vi "Periodic Tasks.vi"(8 "error in":errorcluster) -> ()   [LabVIEW 2020]
doc: "This VI runs in parallel to other tasks. It can contain as many user-defined periodic loops as you need. These can carry out PID or other sorts of timed response."
uses:
  <vilib>/Rock Robotics/WPI/ThirdParty/Phoenix-LabVIEW/Motor Controller/Controls/CTRE_Phoenix_MotorControl_ControlMode.ctl
  <vilib>/Rock Robotics/WPI/DriverStation/WPI_DriverStationRobotMode2.ctl
  <vilib>/Rock Robotics/WPI/Utilities/WPI_GetSetVariantRefNum.vi
  <vilib>/Rock Robotics/Network Tables/NT Write Numeric Array.vi
  Robot Global Data.vi
  <vilib>/Rock Robotics/Network Tables/NT Write Boolean Array.vi
  <vilib>/Rock Robotics/Network Tables/NT Write Number.vi
  <vilib>/Rock Robotics/Network Tables/NT Write Boolean.vi
  <vilib>/Rock Robotics/WPI/RobotDrive/WPI_RobotDriveMecanumDrive_Cartesian.vi
panel:
  out "Slow Speed ON":bool
  out "Backwards ON":bool
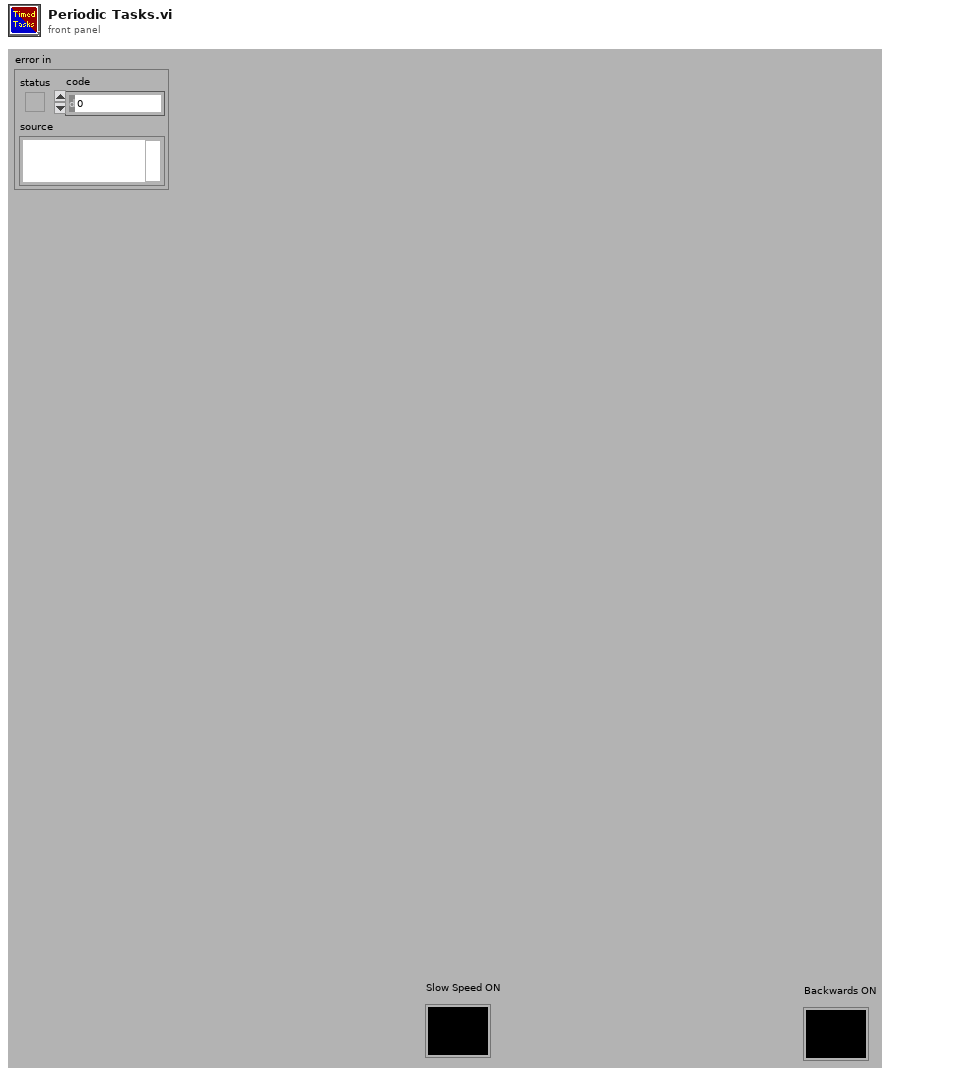
[diagram p1: front panel]
types:
  T1 = typedef "WPI_MotorControlDeviceRef.ctl" = cluster{"DeviceStatus":errorcluster, "Type":T2, "PWM":cluster{"PWM Channel":T3, "DeadBand":T4}, "CAN":cluster{"Device Number":u8, "SetOutput VI Ref":variant, "GetOutput VI Ref":variant, "Enable VI Ref":variant, "Disable VI Ref":variant, "Data":variant}, "Invert":bool, "DIO PWM":cluster{"PWM \"Enable\" Channel":T3, "DIOChannel":T5, "PWM Rate":dbl}}
  T2 = typedef "WPI_MotorControlType.ctl" = enum16{"PWM", "CAN", "DIO PWM"}
  T3 = typedef "FPGA_DIOPWMChannel.ctl" = enum8{"PWM 0", "PWM 1", "PWM 2", "PWM 3", "PWM 4", "PWM 5", "PWM 6", "PWM 7", "PWM 8", "PWM 9", "PWM MXP 0", "PWM MXP 1", "PWM MXP 2", "PWM MXP 3", "PWM MXP 4", "PWM MXP 5", "PWM MXP 6", "PWM MXP 7", "PWM MXP 8", "PWM MXP 9", "Invalid"}
  T4 = typedef "WPI_PWMDeadband.ctl" = cluster{"Name":string, "maxPositivePwm":i32, "minPositivePwm":i32, "centerPwm":i32, "maxNegativePwm":i32, "minNegativePwm":i32, "angularRange":u16}
  T5 = typedef "FPGA_DIOChannel.ctl" = enum8{"DIO 0", "DIO 1", "DIO 2", "DIO 3", "DIO 4", "DIO 5", "DIO 6", "DIO 7", "DIO 8", "DIO 9", "DIO MXP 0", "DIO MXP 1", "DIO MXP 2", "DIO MXP 3", "DIO MXP 4", "DIO MXP 5", "DIO MXP 6", "DIO MXP 7", "DIO MXP 8", "DIO MXP 9", "DIO MXP 10", "DIO MXP 11", "DIO MXP 12", "DIO MXP 13", "DIO MXP 14", "DIO MXP 15", "SPI Port CS1", "SPI Port CS2", "SPI Port CS3", "SPI Port MISO", "SPI Port MOSI", "Invalid"}
  T6 = typedef "WPI_JoystickDevRef.ctl" = cluster{"Device":T7}
  T7 = typedef "WPI_JoystickDeviceEnum.ctl" = enum16{"USB 0", "USB 1", "USB 2", "USB 3", "USB 4", "USB 5"}
  T8 = typedef "WPI_RobotDriveDevRef.ctl" = cluster{"DevStatus":errorcluster, "Motors[]":T1[], "Square Inputs":bool, "Max Output":dbl}
  T9 = typedef "WPI_ServoDeviceRef.ctl" = cluster{"DeviceStatus":errorcluster, "PWM Channel":T3, "DeadBand":T4}
  T10 = typedef "WPI_DriverStationRobotMode2.ctl" = enum16{"Autonomous Disabled", "Autonomous Enabled", "Teleop Disabled", "Teleop Enabled", "Disconnected", "Finish", "Test Disabled", "Test Enabled", "Emergency Stopped"}
  T11 = typedef "CTRE_Phoenix_MotorControl_ControlMode.ctl" = u16
  T12 = typedef "WPI_GyroDevRef.ctl" = cluster{"DevStatus":errorcluster, "Analog Channel":T13, "Gain (VoltsPerDegree/Second)":dbl, "Gyro Type":enum16{"Analog", "XRS450"}, "Handle":i32, "SPI Bus":T14, "Device Found":bool, "Sample Rate":dbl, "Calibrate On Open":bool, "Offset":dbl}
  T13 = typedef "FPGA_AIChannel.ctl" = enum8{"AI 0", "AI 1", "AI 2", "AI 3", "AI MXP 0", "AI MXP 1", "AI MXP 2", "AI MXP 3", "Invalid"}
  T14 = typedef "spi_bus.ctl" = enum16{"SPI On-Board, CS0", "SPI On-Board, CS1", "SPI On-Board, CS2", "SPI On-Board, CS3", "SPI MXP", "Invalid"}
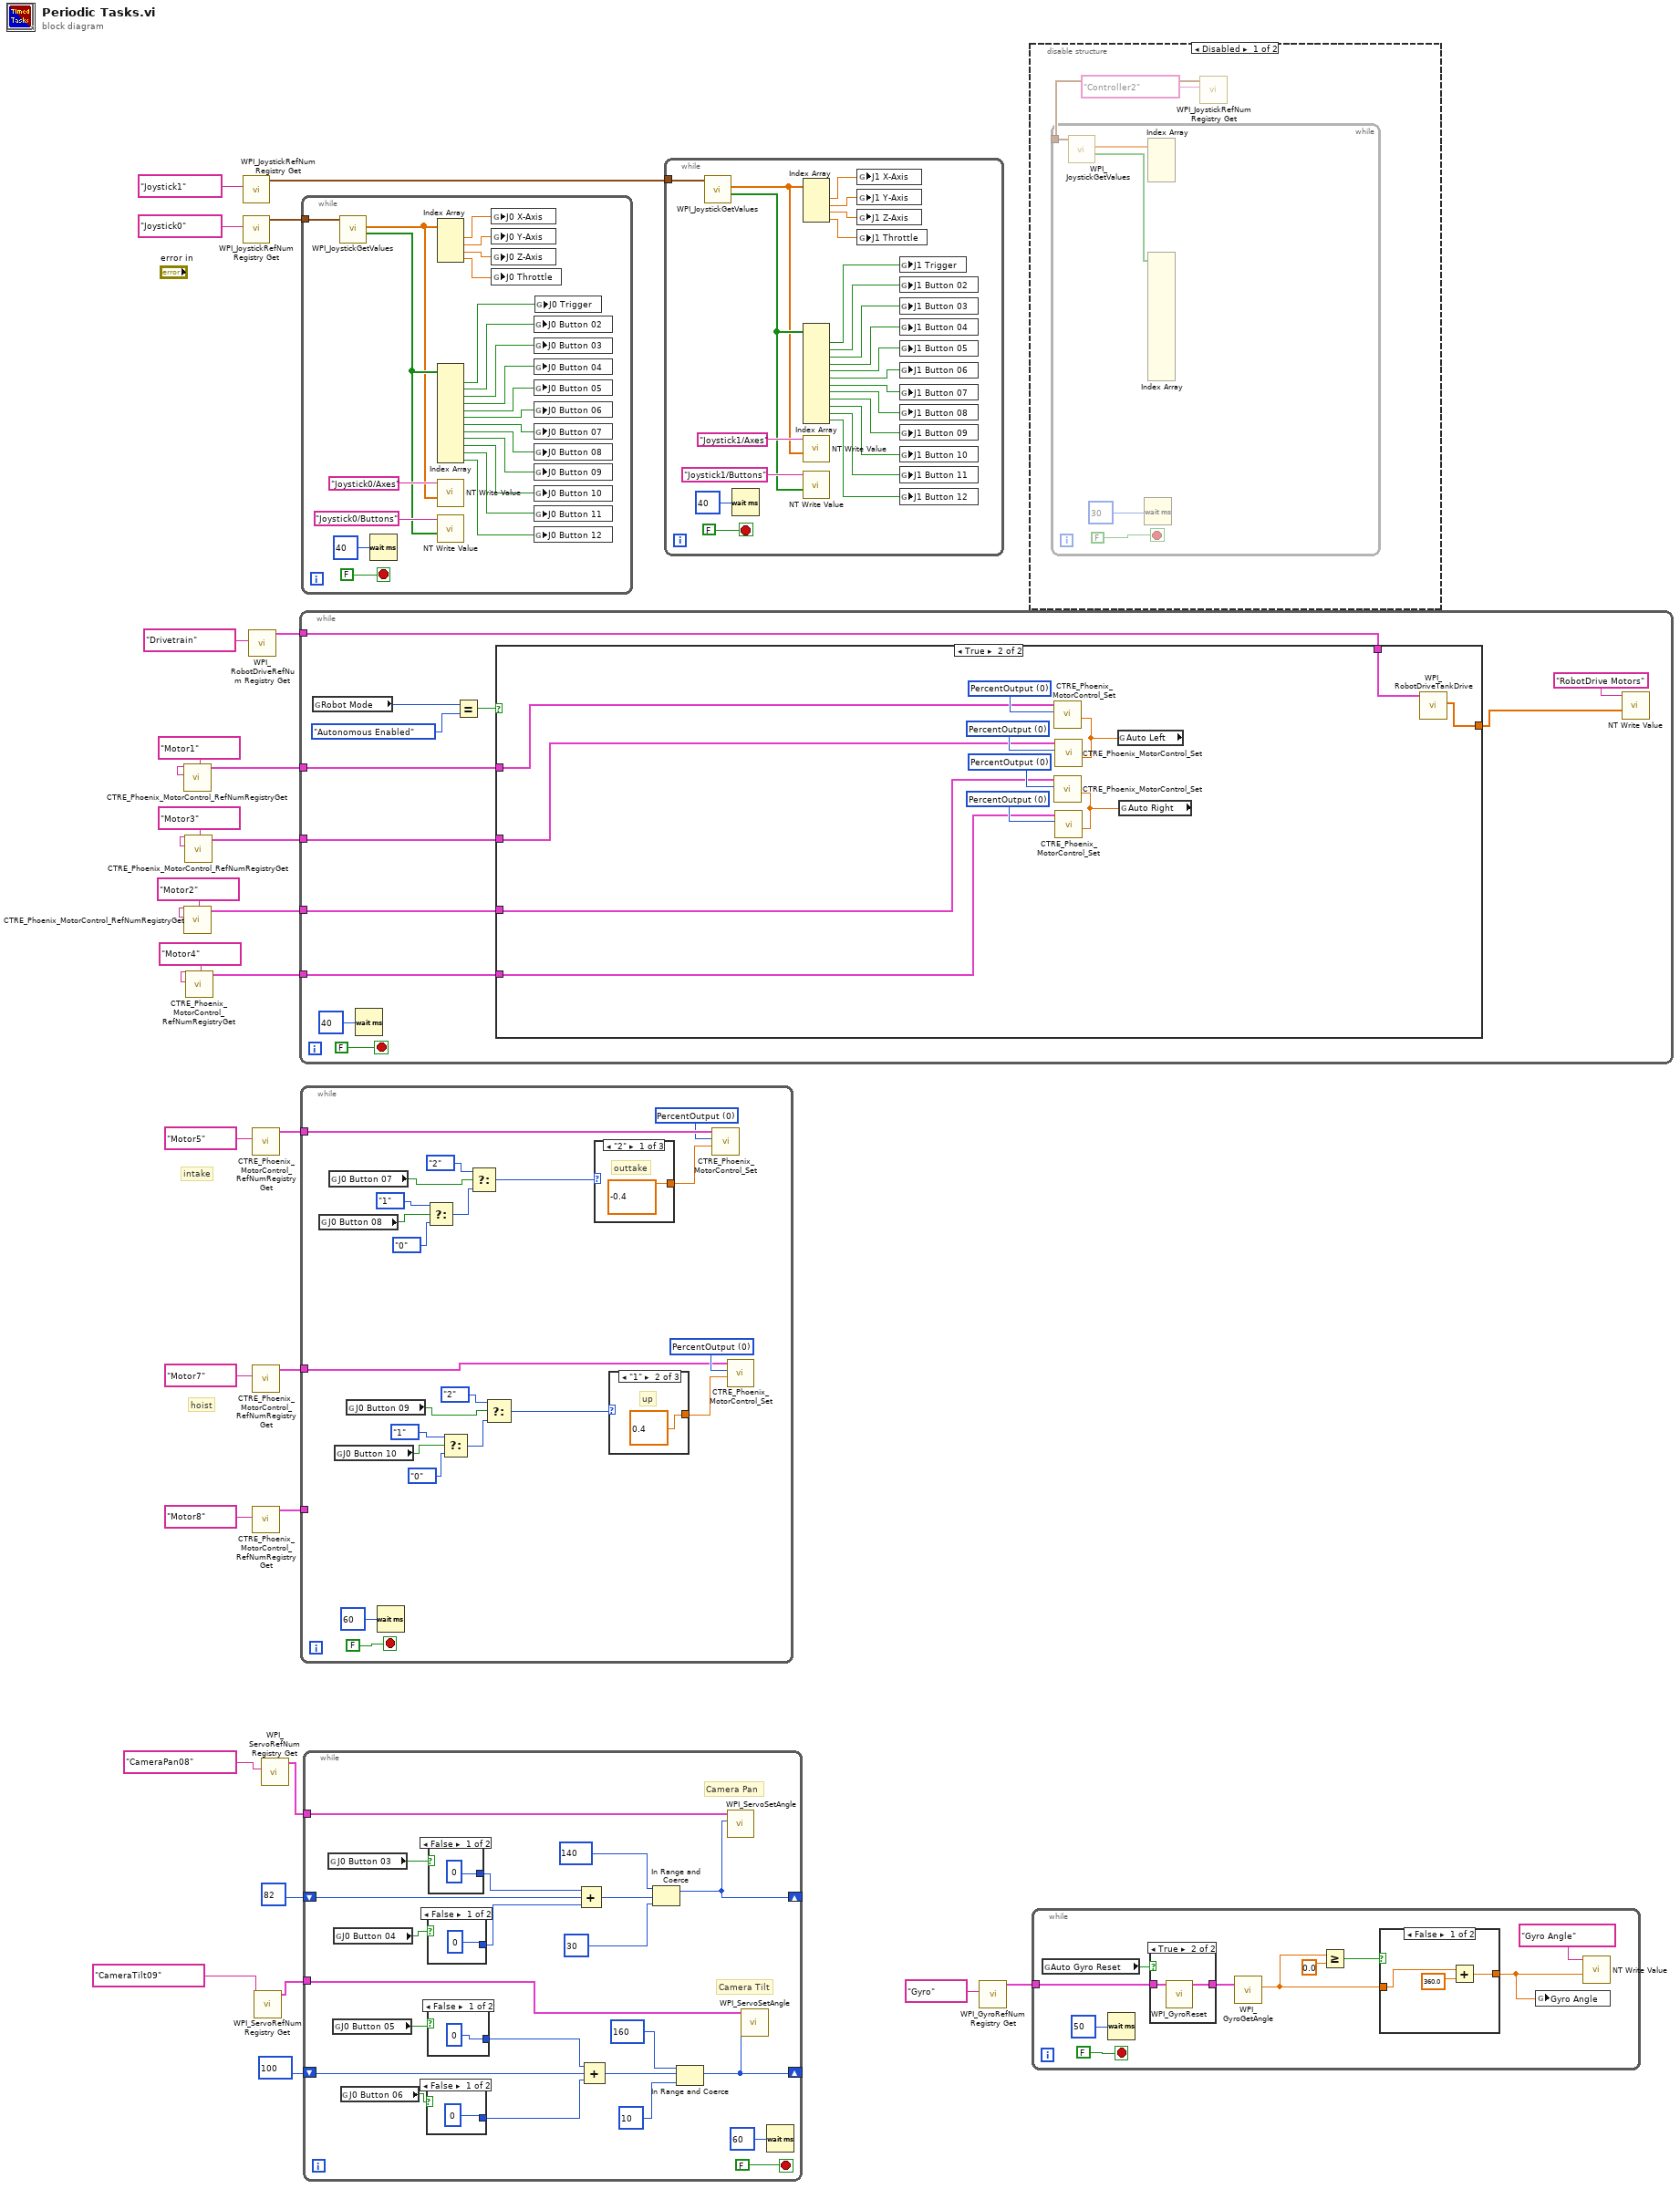
[diagram p0: block diagram]
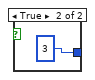
[diagram p4: hidden frame]
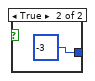
[diagram p5: hidden frame]
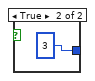
[diagram p6: hidden frame]
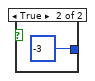
[diagram p7: hidden frame]
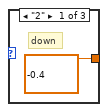
[diagram p9: hidden frame]
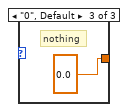
[diagram p10: hidden frame]
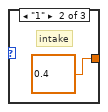
[diagram p11: hidden frame]
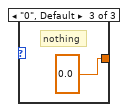
[diagram p12: hidden frame]
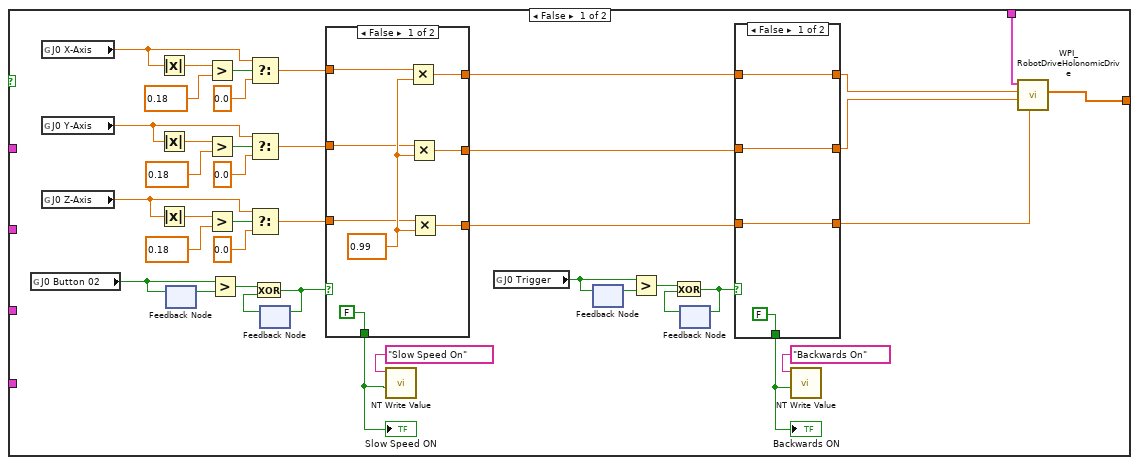
[diagram p13: hidden frame]
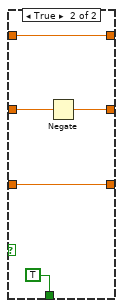
[diagram p14: hidden frame]
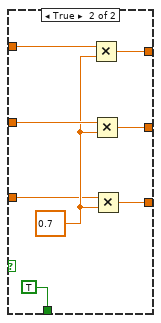
[diagram p15: hidden frame]
diagram:
  # "hoist"
  # "intake"
  n1 = call <vilib>:"CTRE_Phoenix_MotorControl_RefNumRegistryGet.vi"("refnum name"="Motor1") -> ("PhoenixMotorControlDevRef"=w1:T1)  [unwired: 9 in, 1 out]
  n2 = call <vilib>:"CTRE_Phoenix_MotorControl_RefNumRegistryGet.vi"("refnum name"="Motor2") -> ("PhoenixMotorControlDevRef"=w3:T1)  [unwired: 9 in, 1 out]
  n3 = call <vilib>:"CTRE_Phoenix_MotorControl_RefNumRegistryGet.vi"("refnum name"="Motor3") -> ("PhoenixMotorControlDevRef"=w2:T1)  [unwired: 9 in, 1 out]
  n4 = call <vilib>:"CTRE_Phoenix_MotorControl_RefNumRegistryGet.vi"("refnum name"="Motor4") -> ("PhoenixMotorControlDevRef"=w4:T1)  [unwired: 9 in, 1 out]
  n5 = call <vilib>:"WPI_JoystickRefNum Registry Get.vi"("refnum name"="Joystick1") -> ("JoystickDevRef"=w24:T6)  [unwired: 1 in, 9 out]
  n6 = call <vilib>:"WPI_JoystickRefNum Registry Get.vi"("refnum name"="Joystick0") -> ("JoystickDevRef"=w26:T6)  [unwired: 1 in, 9 out]
  n7 = call <vilib>:"WPI_RobotDriveRefNum Registry Get.vi"("refnum name"="Drivetrain") -> ("RobotDriveDevRef"=w9:T8)  [unwired: 9 in, 1 out]
  n8 = call <vilib>:"CTRE_Phoenix_MotorControl_RefNumRegistryGet.vi"("refnum name"="Motor5") -> ("PhoenixMotorControlDevRef"=w20:T1)  [unwired: 9 in, 1 out]
  n9 = call <vilib>:"CTRE_Phoenix_MotorControl_RefNumRegistryGet.vi"("refnum name"="Motor7") -> ("PhoenixMotorControlDevRef"=w19:T1)  [unwired: 9 in, 1 out]
  n10 = call <vilib>:"CTRE_Phoenix_MotorControl_RefNumRegistryGet.vi"("refnum name"="Motor8") -> ("PhoenixMotorControlDevRef"=w18:T1)  [unwired: 9 in, 1 out]
  n11 = call <vilib>:"WPI_ServoRefNum Registry Get.vi"("refnum name"="CameraTilt09") -> ("ServoDeviceRef"=w14:T9)  [unwired: 9 in, 1 out]
  n12 = call <vilib>:"WPI_ServoRefNum Registry Get.vi"("refnum name"="CameraPan08") -> ("ServoDeviceRef"=w15:T9)  [unwired: 9 in, 1 out]
  n13 = while {
    tunnel: w9 -> [w34]
    tunnel: w4 -> [w32]
    tunnel: w3 -> [w31]
    tunnel: w2 -> [w30]
    tunnel: w1 -> [w29]
    stop <- FALSE stop-if-true
    n14 = global read "Robot Global Data.vi" "Robot Mode"() -> (w38:T10)
    n15 = Wait (ms)(milliseconds to wait=u32 40) -> ()  [unwired: 1 out]
    n16 = Equal?(x=w38, y=WPI_DriverStationRobotMode2."Autonomous Enabled" ("Robot Mode")) -> (x = y?=w36:bool)
    n17 = case shown="True" w36 {
      tunnel: w34 -> [w42 w110]
      tunnel: [w41 w111] -> w33
      tunnel: w32 -> [_ w106]
      tunnel: w31 -> [_ w109]
      tunnel: w30 -> [_ w108]
      tunnel: w29 -> [_ w107]
      frame False {
        n18 = global read "Robot Global Data.vi" "J0 Button 02"() -> (w55:bool)
        n19 = global read "Robot Global Data.vi" "J0 X-Axis"() -> (w59:dbl)
        n20 = global read "Robot Global Data.vi" "J0 Y-Axis"() -> (w58:dbl)
        n21 = global read "Robot Global Data.vi" "J0 Z-Axis"() -> (w57:dbl)
        n22 = Absolute Value(x=w59) -> (abs(x)=w74:dbl)
        n23 = Absolute Value(x=w58) -> (abs(x)=w76:dbl)
        n24 = Absolute Value(x=w57) -> (abs(x)=w68:dbl)
        n25 = feedback #1() -> (w79:bool)  [unwired: 1 in]
        n26 = feedback-in #1(w55) -> ()
        n27 = Greater?(x=w74, y=0.18) -> (0:w75:bool)
        n28 = Greater?(x=w76, y=0.18) -> (0:w77:bool)
        n29 = Greater?(x=w68, y=0.18) -> (0:w69:bool)
        n30 = Greater?(x=w55, y=w79) -> (0:w78:bool)
        n31 = Select(t=w59, s=w75, f=0.0) -> (s? t:f=w60:dbl)
        n32 = Select(t=w58, s=w77, f=0.0) -> (s? t:f=w61:dbl)
        n33 = Select(t=w57, s=w69, f=0.0) -> (s? t:f=w62:dbl)
        n34 = feedback #2() -> (w80:bool)  [unwired: 1 in]
        n35 = Exclusive Or(1:w80, 2:w78) -> (0:w56:bool)
        n36 = feedback-in #2(w56) -> ()
        n37 = case shown="False" w56 {
          tunnel: w60 -> [w96 w105]
          tunnel: w61 -> [w95 w104]
          tunnel: [w93 w103] -> w48
          tunnel: [w92 w102] -> w47
          tunnel: w62 -> [w94 w100]
          tunnel: [w91 w99] -> w46
          tunnel: [FALSE ("Boolean") TRUE ("Boolean")] -> w54
          frame False {
            w97 = 0.99 ("y")
            n38 = Multiply(x=w96, y=w97) -> (x*y=w93:dbl)
            n39 = Multiply(x=w95, y=w97) -> (x*y=w92:dbl)
            n40 = Multiply(x=w94, y=w97) -> (x*y=w91:dbl)
          }
          frame True {
            w101 = 0.7 ("y")
            n41 = Multiply(x=w105, y=w101) -> (x*y=w103:dbl)
            n42 = Multiply(x=w104, y=w101) -> (x*y=w102:dbl)
            n43 = Multiply(x=w100, y=w101) -> (x*y=w99:dbl)
          }
        }
        "Slow Speed ON" <- w54
        n44 = call-poly <vilib>:"NT Write Value.vi"("Boolean"=w54, "Name"="Slow Speed On") -> ()  [unwired: 9 in, 1 out]
        n45 = global read "Robot Global Data.vi" "J0 Trigger"() -> (w53:bool)
        n46 = feedback #3() -> (w52:bool)  [unwired: 1 in]
        n47 = feedback-in #3(w53) -> ()
        n48 = Greater?(x=w53, y=w52) -> (0:w63:bool)
        n49 = feedback #4() -> (w51:bool)  [unwired: 1 in]
        n50 = Exclusive Or(1:w51, 2:w63) -> (0:w50:bool)
        n51 = feedback-in #4(w50) -> ()
        n52 = case shown="False" w50 {
          tunnel: w47 -> [w83 w88]
          tunnel: w48 -> [w81 w86]
          tunnel: [w83 w87] -> w44
          tunnel: [w81 w86] -> w43
          tunnel: w46 -> [w82 w85]
          tunnel: [w82 w85] -> w45
          tunnel: [FALSE ("Boolean") TRUE ("Boolean")] -> w49
          frame False {
          }
          frame True {
            n53 = Negate(x=w88) -> (-x=w87:dbl)
          }
        }
        "Backwards ON" <- w49
        n54 = call-poly <vilib>:"NT Write Value.vi"("Boolean"=w49, "Name"="Backwards On") -> ()  [unwired: 9 in, 1 out]
        n55 = call-poly <vilib>:"WPI_RobotDriveHolonomicDrive.vi"("Rotation"=w45, "Y"=w44, "X"=w43, "RobotDriveDevRef"=w42) -> ("Motor Values"=w41:dbl[])  [unwired: 5 in, 2 out]
      }
      frame True {
        w114 = T11 0 items=["PercentOutput"=0, "Position"=1, "Velocity"=2, "Current"=3, "Follower"=5, "MotionProfile"=6, "MotionMagic"=7, "MotionProfileArc"=10, "Disabled"=15] ("Control Mode")
        w115 = T11 0 items=["PercentOutput"=0, "Position"=1, "Velocity"=2, "Current"=3, "Follower"=5, "MotionProfile"=6, "MotionMagic"=7, "MotionProfileArc"=10, "Disabled"=15] ("Control Mode")
        w116 = T11 0 items=["PercentOutput"=0, "Position"=1, "Velocity"=2, "Current"=3, "Follower"=5, "MotionProfile"=6, "MotionMagic"=7, "MotionProfileArc"=10, "Disabled"=15] ("Control Mode")
        w117 = T11 0 items=["PercentOutput"=0, "Position"=1, "Velocity"=2, "Current"=3, "Follower"=5, "MotionProfile"=6, "MotionMagic"=7, "MotionProfileArc"=10, "Disabled"=15] ("Control Mode")
        n56 = global read "Robot Global Data.vi" "Auto Left"() -> (w113:dbl)
        n57 = call <vilib>:"CTRE_Phoenix_MotorControl_Set.vi"("Output"=w113, "Control Mode"=w117, "PhoenixMotorControlDevRef"=w107) -> ()  [unwired: 7 in, 2 out]
        n58 = call <vilib>:"CTRE_Phoenix_MotorControl_Set.vi"("Output"=w113, "Control Mode"=w116, "PhoenixMotorControlDevRef"=w108) -> ()  [unwired: 7 in, 2 out]
        n59 = global read "Robot Global Data.vi" "Auto Right"() -> (w112:dbl)
        n60 = call <vilib>:"CTRE_Phoenix_MotorControl_Set.vi"("Output"=w112, "Control Mode"=w115, "PhoenixMotorControlDevRef"=w109) -> ()  [unwired: 7 in, 2 out]
        n61 = call <vilib>:"CTRE_Phoenix_MotorControl_Set.vi"("Output"=w112, "Control Mode"=w114, "PhoenixMotorControlDevRef"=w106) -> ()  [unwired: 7 in, 2 out]
        n62 = call <vilib>:"WPI_RobotDriveTankDrive.vi"("RobotDriveDevRef"=w110) -> ("Motor Values"=w111:dbl[])  [unwired: 8 in, 2 out]
      }
    }
    n63 = call-poly <vilib>:"NT Write Value.vi"("Numeric Array"=w33, "Name"="RobotDrive Motors") -> ()  [unwired: 9 in, 1 out]
  }
  n64 = while {
    tunnel: w20 -> [w139]
    tunnel: w19 -> [w120]
    tunnel: w18 -> [_]
    stop <- FALSE stop-if-true
    w128 = T11 0 items=["PercentOutput"=0, "Position"=1, "Velocity"=2, "Current"=3, "Follower"=5, "MotionProfile"=6, "MotionMagic"=7, "MotionProfileArc"=10, "Disabled"=15] ("Control Mode")
    w138 = T11 0 items=["PercentOutput"=0, "Position"=1, "Velocity"=2, "Current"=3, "Follower"=5, "MotionProfile"=6, "MotionMagic"=7, "MotionProfileArc"=10, "Disabled"=15] ("Control Mode")
    n65 = global read "Robot Global Data.vi" "J0 Button 08"() -> (w118:bool)
    n66 = global read "Robot Global Data.vi" "J0 Button 07"() -> (w133:bool)
    n67 = global read "Robot Global Data.vi" "J0 Button 10"() -> (w119:bool)
    n68 = global read "Robot Global Data.vi" "J0 Button 09"() -> (w125:bool)
    n69 = Wait (ms)(milliseconds to wait=u32 60) -> ()  [unwired: 1 out]
    n70 = Select(t=enum16{"2", "1", "0", ""}."1", s=w118, f=enum16{"2", "1", "0", ""}."0") -> (s? t:f=w134:enum16{"2", "1", "0", ""})
    n71 = Select(t=enum16{"2", "1", "0", ""}."1", s=w119, f=enum16{"2", "1", "0", ""}."0") -> (s? t:f=w126:enum16{"2", "1", "0", ""})
    n72 = Select(t=enum16{"2", "1", "0", ""}."2", s=w133, f=w134) -> (s? t:f=w132:enum16{"2", "1", "0", ""})
    n73 = Select(t=enum16{"2", "1", "0", ""}."2", s=w125, f=w126) -> (s? t:f=w124:enum16{"2", "1", "0", ""})
    n74 = case shown="\"2\"" w132 {
      tunnel: [-0.4 0.4 0.0] -> w137
      frame "2" {
        # "outtake"
      }
      frame "1" {
        # "intake"
      }
      frame "0", Default {
        # "nothing"
      }
    }
    n75 = case shown="\"1\"" w124 {
      tunnel: [-0.4 0.4 0.0] -> w127
      frame "2" {
        # "down"
      }
      frame "1" {
        # "up"
      }
      frame "0", Default {
        # "nothing"
      }
    }
    n76 = call <vilib>:"CTRE_Phoenix_MotorControl_Set.vi"("Output"=w137, "Control Mode"=w138, "PhoenixMotorControlDevRef"=w139) -> ()  [unwired: 7 in, 2 out]
    n77 = call <vilib>:"CTRE_Phoenix_MotorControl_Set.vi"("Output"=w127, "Control Mode"=w128, "PhoenixMotorControlDevRef"=w120) -> ()  [unwired: 7 in, 2 out]
  }
  n78 = while {
    tunnel: w26 -> [w166]
    stop <- FALSE stop-if-true
    n79 = call <vilib>:"WPI_JoystickGetValues.vi"("JoystickDevRef"=w166) -> ("Buttons"=w147:bool[], "Axes"=w146:dbl[])  [unwired: 6 in, 3 out]
    n80 = Wait (ms)(milliseconds to wait=u32 40) -> ()  [unwired: 1 out]
    n81 = Index Array(array=w146) -> (element #1=w165:dbl, element #2=w164:dbl, element #3=w163:dbl, element #4=w162:dbl)  [unwired: 4 in]
    n82 = Index Array(array=w147) -> (element #1=w161:bool, element #2=w160:bool, element #3=w159:bool, element #4=w158:bool, element #5=w157:bool, element #6=w156:bool, element #7=w155:bool, element #8=w154:bool, element #9=w153:bool, element #10=w152:bool, element #11=w151:bool, element #12=w150:bool)  [unwired: 12 in]
    n83 = call-poly <vilib>:"NT Write Value.vi"("Numeric Array"=w146, "Name"="Joystick0/Axes") -> ()  [unwired: 9 in, 1 out]
    n84 = call-poly <vilib>:"NT Write Value.vi"("Boolean Array"=w147, "Name"="Joystick0/Buttons") -> ()  [unwired: 9 in, 1 out]
    n85 = global write "Robot Global Data.vi" "J0 X-Axis"(w165) -> ()
    n86 = global write "Robot Global Data.vi" "J0 Y-Axis"(w164) -> ()
    n87 = global write "Robot Global Data.vi" "J0 Z-Axis"(w163) -> ()
    n88 = global write "Robot Global Data.vi" "J0 Throttle"(w162) -> ()
    n89 = global write "Robot Global Data.vi" "J0 Button 02"(w160) -> ()
    n90 = global write "Robot Global Data.vi" "J0 Button 03"(w159) -> ()
    n91 = global write "Robot Global Data.vi" "J0 Button 04"(w158) -> ()
    n92 = global write "Robot Global Data.vi" "J0 Button 05"(w157) -> ()
    n93 = global write "Robot Global Data.vi" "J0 Button 06"(w156) -> ()
    n94 = global write "Robot Global Data.vi" "J0 Button 07"(w155) -> ()
    n95 = global write "Robot Global Data.vi" "J0 Button 08"(w154) -> ()
    n96 = global write "Robot Global Data.vi" "J0 Button 09"(w153) -> ()
    n97 = global write "Robot Global Data.vi" "J0 Button 10"(w152) -> ()
    n98 = global write "Robot Global Data.vi" "J0 Button 11"(w151) -> ()
    n99 = global write "Robot Global Data.vi" "J0 Button 12"(w150) -> ()
    n100 = global write "Robot Global Data.vi" "J0 Trigger"(w161) -> ()
  }
  n101 = while {
    tunnel: w15 -> [w190]
    tunnel: w14 -> [w189]
    shift-right: [w177] -> _
    shift-left: 82 -> [w170]
    shift-right: [w169] -> _
    shift-left: 100 -> [w186]
    stop <- FALSE stop-if-true
    # "Camera Tilt"
    # "Camera Pan"
    n102 = global read "Robot Global Data.vi" "J0 Button 03"() -> (w173:bool)
    n103 = global read "Robot Global Data.vi" "J0 Button 05"() -> (w175:bool)
    n104 = global read "Robot Global Data.vi" "J0 Button 04"() -> (w174:bool)
    n105 = global read "Robot Global Data.vi" "J0 Button 06"() -> (w176:bool)
    n106 = case shown="False" w176 {
      tunnel: [0 3] -> w185
      frame False {
      }
      frame True {
      }
    }
    n107 = case shown="False" w174 {
      tunnel: [0 3] -> w187
      frame False {
      }
      frame True {
      }
    }
    n108 = case shown="False" w175 {
      tunnel: [0 -3] -> w184
      frame False {
      }
      frame True {
      }
    }
    n109 = case shown="False" w173 {
      tunnel: [0 -3] -> w188
      frame False {
      }
      frame True {
      }
    }
    n110 = Compound Arithmetic op=ADD(w188, w170, w187) -> (w181:i32)
    n111 = Compound Arithmetic op=ADD(w184, w186, w185) -> (w178:i32)
    n112 = In Range and Coerce(upper limit=140, x=w181, lower limit=30) -> (coerced(x)=w177:i32)  [unwired: 1 out]
    n113 = In Range and Coerce(upper limit=160, x=w178, lower limit=10) -> (coerced(x)=w169:i32)  [unwired: 1 out]
    n114 = call <vilib>:"WPI_ServoSetAngle.vi"("Angle"=w177, "ServoDeviceRef"=w190) -> ()  [unwired: 8 in, 2 out]
    n115 = call <vilib>:"WPI_ServoSetAngle.vi"("Angle"=w169, "ServoDeviceRef"=w189) -> ()  [unwired: 8 in, 2 out]
    n116 = Wait (ms)(milliseconds to wait=u32 60) -> ()  [unwired: 1 out]
  }
  n117 = while {
    tunnel: w24 -> [w219]
    stop <- FALSE stop-if-true
    n118 = call <vilib>:"WPI_JoystickGetValues.vi"("JoystickDevRef"=w219) -> ("Buttons"=w200:bool[], "Axes"=w199:dbl[])  [unwired: 6 in, 3 out]
    n119 = Wait (ms)(milliseconds to wait=u32 40) -> ()  [unwired: 1 out]
    n120 = Index Array(array=w199) -> (element #1=w218:dbl, element #2=w217:dbl, element #3=w216:dbl, element #4=w215:dbl)  [unwired: 4 in]
    n121 = Index Array(array=w200) -> (element #1=w214:bool, element #2=w213:bool, element #3=w212:bool, element #4=w211:bool, element #5=w210:bool, element #6=w209:bool, element #7=w208:bool, element #8=w207:bool, element #9=w206:bool, element #10=w205:bool, element #11=w204:bool, element #12=w203:bool)  [unwired: 12 in]
    n122 = call-poly <vilib>:"NT Write Value.vi"("Numeric Array"=w199, "Name"="Joystick1/Axes") -> ()  [unwired: 9 in, 1 out]
    n123 = call-poly <vilib>:"NT Write Value.vi"("Boolean Array"=w200, "Name"="Joystick1/Buttons") -> ()  [unwired: 9 in, 1 out]
    n124 = global write "Robot Global Data.vi" "J1 X-Axis"(w218) -> ()
    n125 = global write "Robot Global Data.vi" "J1 Y-Axis"(w217) -> ()
    n126 = global write "Robot Global Data.vi" "J1 Z-Axis"(w216) -> ()
    n127 = global write "Robot Global Data.vi" "J1 Throttle"(w215) -> ()
    n128 = global write "Robot Global Data.vi" "J1 Trigger"(w214) -> ()
    n129 = global write "Robot Global Data.vi" "J1 Button 02"(w213) -> ()
    n130 = global write "Robot Global Data.vi" "J1 Button 03"(w212) -> ()
    n131 = global write "Robot Global Data.vi" "J1 Button 04"(w211) -> ()
    n132 = global write "Robot Global Data.vi" "J1 Button 05"(w210) -> ()
    n133 = global write "Robot Global Data.vi" "J1 Button 06"(w209) -> ()
    n134 = global write "Robot Global Data.vi" "J1 Button 07"(w208) -> ()
    n135 = global write "Robot Global Data.vi" "J1 Button 08"(w207) -> ()
    n136 = global write "Robot Global Data.vi" "J1 Button 09"(w206) -> ()
    n137 = global write "Robot Global Data.vi" "J1 Button 10"(w205) -> ()
    n138 = global write "Robot Global Data.vi" "J1 Button 11"(w204) -> ()
    n139 = global write "Robot Global Data.vi" "J1 Button 12"(w203) -> ()
  }
  n140 = call <vilib>:"WPI_GyroRefNum Registry Get.vi"("refnum name"="Gyro") -> ("GyroDevRef"=w12:T12)  [unwired: 9 in, 1 out]
  n141 = disable-structure shown="Disabled" {
    frame Disabled {
      n142 = call <vilib>:"WPI_JoystickRefNum Registry Get.vi"("refnum name"="Controller2") -> ("JoystickDevRef"=w222:T6)  [unwired: 1 in, 9 out]
      n143 = while {
        tunnel: w222 -> [w228]
        stop <- FALSE stop-if-true
        n144 = call <vilib>:"WPI_JoystickGetValues.vi"("JoystickDevRef"=w228) -> ("Buttons"=w224:bool[], "Axes"=w225:dbl[])  [unwired: 6 in, 3 out]
        n145 = Wait (ms)(milliseconds to wait=u32 30) -> ()  [unwired: 1 out]
        n146 = Index Array(array=w225) -> ()  [unwired: 4 in, 4 out]
        n147 = Index Array(array=w224) -> ()  [unwired: 16 in, 16 out]
      }
    }
    frame Enabled {
    }
  }
  n148 = while {
    tunnel: w12 -> [w238]
    stop <- FALSE stop-if-true
    n149 = global read "Robot Global Data.vi" "Auto Gyro Reset"() -> (w236:bool)
    n150 = Wait (ms)(milliseconds to wait=u32 50) -> ()  [unwired: 1 out]
    n151 = case shown="True" w236 {
      tunnel: w238 -> [w243 w245]
      tunnel: [w243 w244] -> w237
      frame False {
      }
      frame True {
        n152 = call <vilib>:"WPI_GyroReset.vi"("GyroDevRef"=w245) -> ("GyroDevRef"=w244:T12)  [unwired: 9 in, 1 out]
      }
    }
    n153 = call <vilib>:"WPI_GyroGetAngle.vi"("GyroDevRef"=w237) -> ("Angle"=w233:dbl)  [unwired: 6 in, 4 out]
    n154 = Greater Or Equal?(x=w233, y=0.0) -> (x >= y?=w231:bool)
    n155 = case shown="False" w231 {
      tunnel: w233 -> [w240 w242]
      tunnel: [w239 w242] -> w229
      frame False {
        n156 = Add(x=w240, y=360.0) -> (x+y=w239:dbl)
      }
      frame True {
      }
    }
    n157 = global write "Robot Global Data.vi" "Gyro Angle"(w229) -> ()
    n158 = call-poly <vilib>:"NT Write Value.vi"("Numeric"=w229, "Name"="Gyro Angle" ("refnum name")) -> ()  [unwired: 9 in, 1 out]
  }
